vi "Destroy Events.vi"(8 "error in (no error)":errorcluster, 11 "LogEngine.lvclass":refnum<class "LogEngine.lvclass">) -> (0 "error out":errorcluster, 3 "LogEngine.lvclass":refnum<class "LogEngine.lvclass">)   [LabVIEW 2017, in "LogEngine.lvclass"]
doc: "Developed by Kevin Thompson\nkevin@thompsonengineering.net\n\nCopyright 2018-2020\nThompson Engineering, LLC"
uses:
  LogEngine.lvclass
  LogEngine.lvclass/LogEngine.ctl
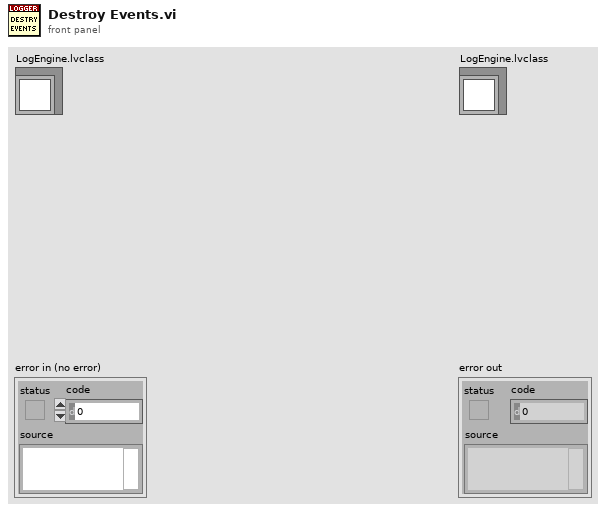
[diagram p1: front panel]
types:
  T1 = typedef "LogEngine.lvclass/TD LogEngine PublicEvents--cluster.ctl" = cluster{"stop process":refnum<user-event>, "LogEngine.AsyncCmd Event":refnum<user-event>, "LogEngine.AsyncMsg Event":refnum<user-event>, "Logger StateChanged Event":refnum<user-event>}
  T2 = cluster{"LogEngine.AsyncCmd Event":refnum<user-event>, "Logger StateChanged Event":refnum<user-event>, "LogEngine.AsyncMsg Event":refnum<user-event>}
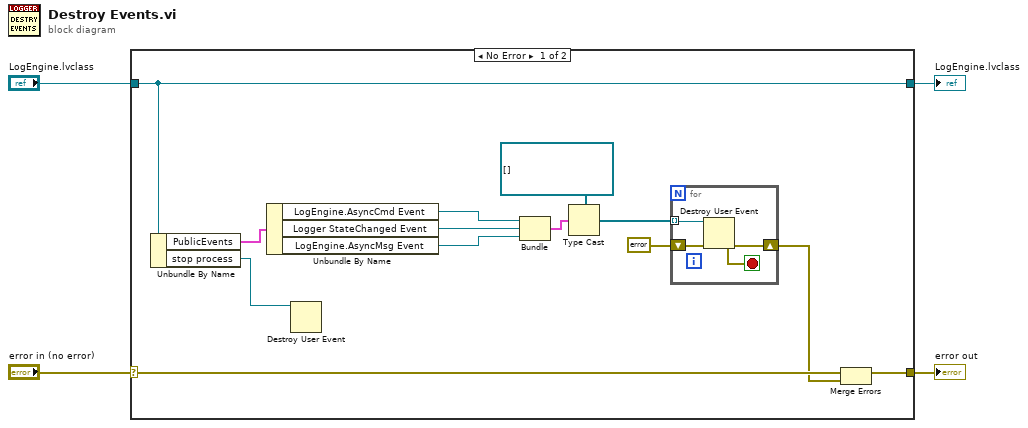
[diagram p0: block diagram]
diagram:
  n1 = case shown="No Error" "error in (no error)" {
    selector: "error in (no error)" -> [w11 w22]
    tunnel: [w12 w22] -> w3
    tunnel: [w17 w21] -> w1
    tunnel: "LogEngine.lvclass" -> [w17 w21]
    frame No Error {
      n2 = Unbundle By Name(w17) -> ("PublicEvents"=w6:T1, "stop process"=w16:refnum<user-event>)
      n3 = Unbundle By Name(w6) -> ("LogEngine.AsyncCmd Event"=w8:refnum<user-event>, "Logger StateChanged Event"=w7:refnum<user-event>, "LogEngine.AsyncMsg Event"=w5:refnum<user-event>)
      n4 = Destroy User Event(user event=w16) -> ()  [unwired: 1 in, 1 out]
      n5 = Bundle("LogEngine.AsyncCmd Event"=w8, "Logger StateChanged Event"=w7, "LogEngine.AsyncMsg Event"=w5) -> (w14:T2)  [unwired: 1 in]
      n6 = Type Cast(type=refnum<user-event>[] [], x=w14) -> (*(type *) &x=w13:refnum<user-event>[])
      n7 = for {
        tunnel: w13 -> [w20] mode=indexing
        shift-right: [w18] -> w10
        shift-left: errorcluster {"status"=FALSE, "code"=0, "source"=""} ("error out") -> [w19]
        stop <- w18 stop-if-true
        n8 = Destroy User Event(user event=w20, error in=w19) -> (error out=w18:errorcluster)
      }
      n9 = Merge Errors(w11, w10) -> (w12:errorcluster)
    }
    frame Error {
    }
  }
  "error out" <- w3
  "LogEngine.lvclass" <- w1
